vi "Get Running Status.vi"(8 "error in (no error)":errorcluster, 11 "Engine Simulation Session in":refnum<class "Engine Simulation Session.lvclass">) -> (0 "error out":errorcluster, 2 "running":bool, 3 "Engine Simulation Session out":refnum<class "Engine Simulation Session.lvclass">)   [LabVIEW 2013, in "Engine Simulation Session.lvclass"]
uses:
  Engine Simulation Session.lvclass
  Engine Simulation Session.lvclass/Engine Simulation Session.ctl
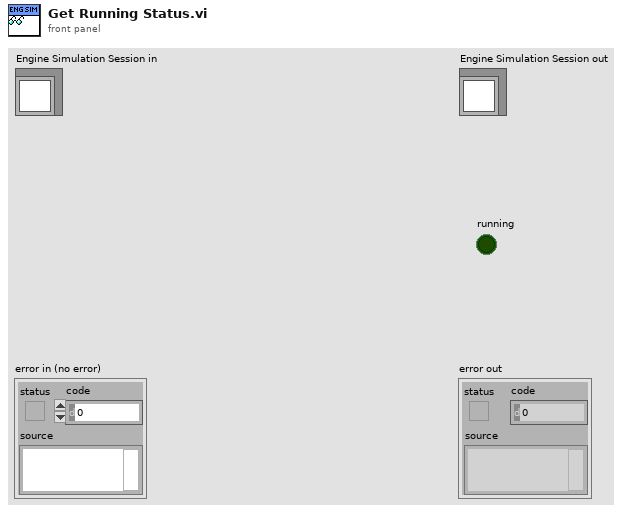
[diagram p1: front panel]
types:
  T1 = typedef "Engine Simulation Session.lvclass/session class private data.ctl" = cluster{"running":bool, "fpga reference":refnum<k20>, "bitfile":path}
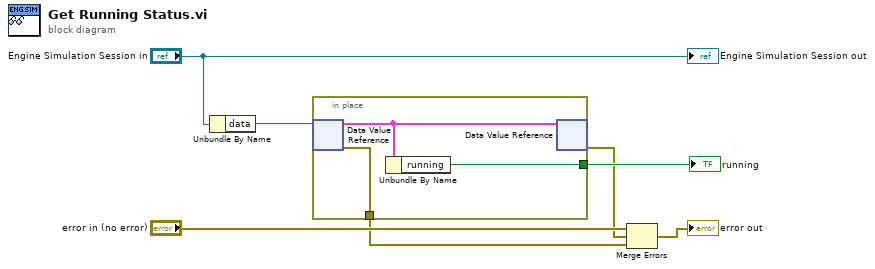
[diagram p0: block diagram]
diagram:
  n1 = Unbundle By Name("Engine Simulation Session in") -> ("data"=w5:refnum<data-value>)
  n2 = in-place {
    in-place-border: [w9] -> w4
    in-place-border: [w8] -> w1
    n3 = in-place-dvr #1(w5) -> (w10:T1, w8:errorcluster)
    n4 = Unbundle By Name(w10) -> ("running"=w9:bool)
    n5 = in-place-dvr #1(w10) -> (w2:errorcluster)  [unwired: 1 out]
  }
  "running" <- w4
  n6 = Merge Errors("error in (no error)", w2, w1) -> (→"error out":errorcluster)
  "Engine Simulation Session out" <- "Engine Simulation Session in"
